vi "Lift.vi"(11 "State":T2(ring)) -> (2 "Lift Motor(Global...)":dbl, 3 "State Out":T2(ring))   [LabVIEW 2014]
uses:
  Global Variables.vi
  <vilib>/addons/control/pid/pid.llb/PID (DBL).vi
  <vilib>/addons/control/pid/NI_PID_pid.lvlib
panel:
  out "Encoder":dbl
  in  "PID gains":T1={"proportional gain (Kc)"=0.006, "integral time (Ti, min)"=0.0, "derivative time (Td, min)"=0.0} {"derivative time (Td, min)" format="%.3f"; "integral time (Ti, min)" format="%.3f"; "proportional gain (Kc)" format="%.3f"}
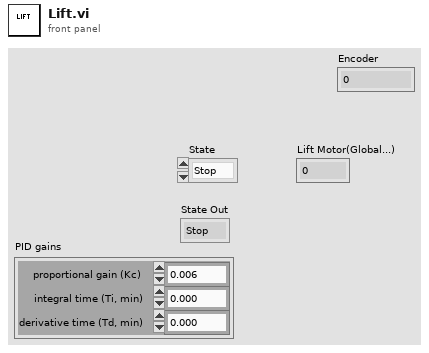
[diagram p1: front panel]
types:
  T1 = cluster{"proportional gain (Kc)":dbl, "integral time (Ti, min)":dbl, "derivative time (Td, min)":dbl}
  T2 = enum16{"Stop", "Three Tote", "Two Tote", "One Tote", "Step", "Top", "Home", "Joystick"}
  T3 = typedef "WPI_EncoderDevRef.ctl" = cluster{"DevStatus":errorcluster, "EncoderIndex":T4, "CounterIndex":T5, "DistancePerCount":dbl, "Decoding Type":T6}
  T4 = typedef "FPGA_EncoderIdx.ctl" = enum8{"Enc 0", "Enc 1", "Enc 2", "Enc 3", "Enc 4", "Enc 5", "Enc 6", "Enc 7", "Invalid"}
  T5 = typedef "FPGA_CounterCtrSystemIndex.ctl" = enum8{"Ctr 0", "Ctr 1", "Ctr 2", "Ctr 3", "Ctr 4", "Ctr 5", "Ctr 6", "Ctr 7", "Invalid"}
  T6 = typedef "WPI_EncoderType.ctl" = enum16{"1x", "2x", "4x"}
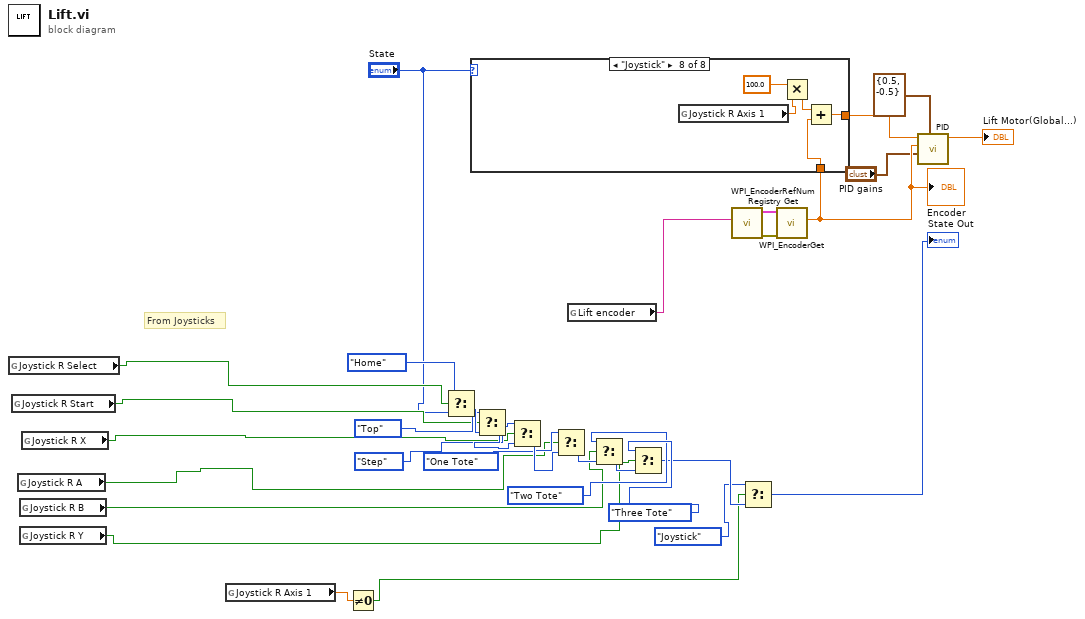
[diagram p0: block diagram]
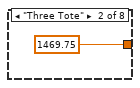
[diagram p3: hidden frame]
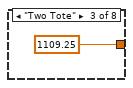
[diagram p4: hidden frame]
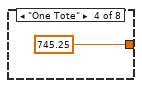
[diagram p5: hidden frame]
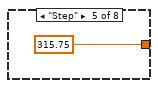
[diagram p6: hidden frame]
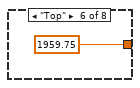
[diagram p7: hidden frame]
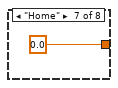
[diagram p8: hidden frame]
diagram:
  # "From Joysticks"
  n1 = global read "Global Variables.vi" "Joystick R Select"() -> (w5:bool)
  n2 = global read "Global Variables.vi" "Joystick R Start"() -> (w4:bool)
  n3 = global read "Global Variables.vi" "Joystick R A"() -> (w9:bool)
  n4 = global read "Global Variables.vi" "Joystick R B"() -> (w8:bool)
  n5 = global read "Global Variables.vi" "Joystick R Y"() -> (w7:bool)
  n6 = global read "Global Variables.vi" "Joystick R X"() -> (w6:bool)
  n7 = global read "Global Variables.vi" "Joystick R Axis 1"() -> (w2:dbl)
  n8 = Not Equal To 0?(x=w2) -> (x != 0?=w3:bool)
  n9 = Select(t=T2."Home" ("State Out"), s=w5, f="State") -> (s? t:f=w29:T2)
  n10 = Select(t=T2."Top" ("State Out"), s=w4, f=w29) -> (s? t:f=w28:T2)
  n11 = Select(t=T2."Step" ("State Out"), s=w6, f=w28) -> (s? t:f=w27:T2)
  n12 = Select(t=T2."One Tote" ("State Out"), s=w9, f=w27) -> (s? t:f=w26:T2)
  n13 = global read "Global Variables.vi" "Lift encoder"() -> (w22:string)
  n14 = Select(t=T2."Two Tote" ("State Out"), s=w8, f=w26) -> (s? t:f=w25:T2)
  n15 = Select(t=T2."Three Tote" ("State Out"), s=w7, f=w25) -> (s? t:f=w11:T2)
  n16 = call <vilib>:"WPI_EncoderRefNum Registry Get.vi"("refnum name"=w22) -> ("error out"=w24:errorcluster, "EncoderDevRef"=w23:T3)  [unwired: 9 in]
  n17 = Select(t=T2."Joystick" ("State Out"), s=w3, f=w11) -> (s? t:f=→"State Out":T2)
  n18 = call <vilib>:"WPI_EncoderGet.vi"("error in (no error)"=w24, "EncoderDevRef"=w23) -> ("Distance"=w20:dbl)  [unwired: 4 in, 5 out]
  "Encoder" <- w20
  n19 = case shown="\"Joystick\"" "State" {
    tunnel: [w32 1469.75 ("setpoint") 1109.25 ("setpoint") 745.25 ("setpoint") 315.75 ("setpoint") 1959.75 ("setpoint") 0.0 ("setpoint") w43] -> w30
    tunnel: w20 -> [w32 _ _ _ _ _ _ w42]
    frame "Stop", Default {
    }
    frame "Three Tote" {
    }
    frame "Two Tote" {
    }
    frame "One Tote" {
    }
    frame "Step" {
    }
    frame "Top" {
    }
    frame "Home" {
    }
    frame "Joystick" {
      n20 = global read "Global Variables.vi" "Joystick R Axis 1"() -> (w39:dbl)
      n21 = Multiply(x=100.0, y=w39) -> (x*y=w41:dbl)
      n22 = Add(x=w41, y=w42) -> (x+y=w43:dbl)
    }
  }
  n23 = call-poly <vilib>:"PID.vi"("output range"=cluster{"output high":dbl, "output low":dbl} {"output high"=0.5, "output low"=-0.5}, "PID gains"="PID gains", "process variable"=w20, "setpoint"=w30) -> ("output"=→"Lift Motor(Global...)":dbl)  [unwired: 6 in, 1 out]
